vi "f1.vi"() -> ()   [LabVIEW 2020]
uses:
  <vilib>/MakerHub/LINX/Public/Peripherals/Analog/Analog Read 1 Chan.vi
  <vilib>/MakerHub/LINX/Public/Peripherals/Digital/Digital Write 1 Chan.vi
  <vilib>/MakerHub/LINX/Public/Peripherals/Analog/Analog Read N Chans.vi
  <vilib>/MakerHub/LINX/Public/Peripherals/Digital/Digital Write N Chans.vi
  <vilib>/MakerHub/LINX/Private/Local IO/LinxAnalogRead.vi
  <vilib>/MakerHub/LINX/Public/Utilities/Check Channel.vi
  <vilib>/MakerHub/LINX/Private/Local IO/LinxDigitalWrite.vi
  <vilib>/MakerHub/LINX/Public/Utilities/Open Serial.vi
  <vilib>/MakerHub/LINX/Private/Utilties/Generate Error.vi
  <vilib>/MakerHub/LINX/LMH-LINX.lvlib
panel:
  out "Voltage":dbl
  in  "stop":bool
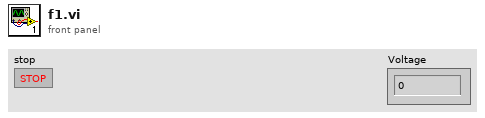
[diagram p1: front panel]
types:
  T1 = typedef "LMH-LINX.lvlib/LINX Ref.ctl" = cluster{"IO":T2, "Interface":T3, "LINX Device Config":T4}
  T2 = typedef "LMH-LINX.lvlib/Platform.ctl" = enum16{"Remote", "Local"}
  T3 = typedef "LMH-LINX.lvlib/Interface.ctl" = enum16{"Serial", "TCP"}
  T4 = typedef "LMH-LINX.lvlib/Device.lvlib/LINX Device Config.ctl" = cluster{"Interface":T3, "COM Port":refnum<visa-resource-name>, "TCP Configuration":T5, "Device Family":u8, "Device ID":u8, "Device Name":string, "TCP Ref":refnum<k5>, "Channels":T6}
  T5 = typedef "LMH-LINX.lvlib/Device.lvlib/TCP Config.ctl" = cluster{"IP Address":string, "Port":u16}
  T6 = typedef "LMH-LINX.lvlib/Channels.ctl" = cluster{"DI":u8[], "DO":u8[], "AI":u8[], "AO":u8[], "PWM":u8[], "QE":u8[], "UART":u8[], "I2C 2":u8[], "SPI":u8[], "CAN":u8[], "Servo":u8[], "AI Ref (V)":dbl, "AI Resolution (Bits)":u8, "AO Ref (V)":dbl, "AO Resolution (Bits)":u8}
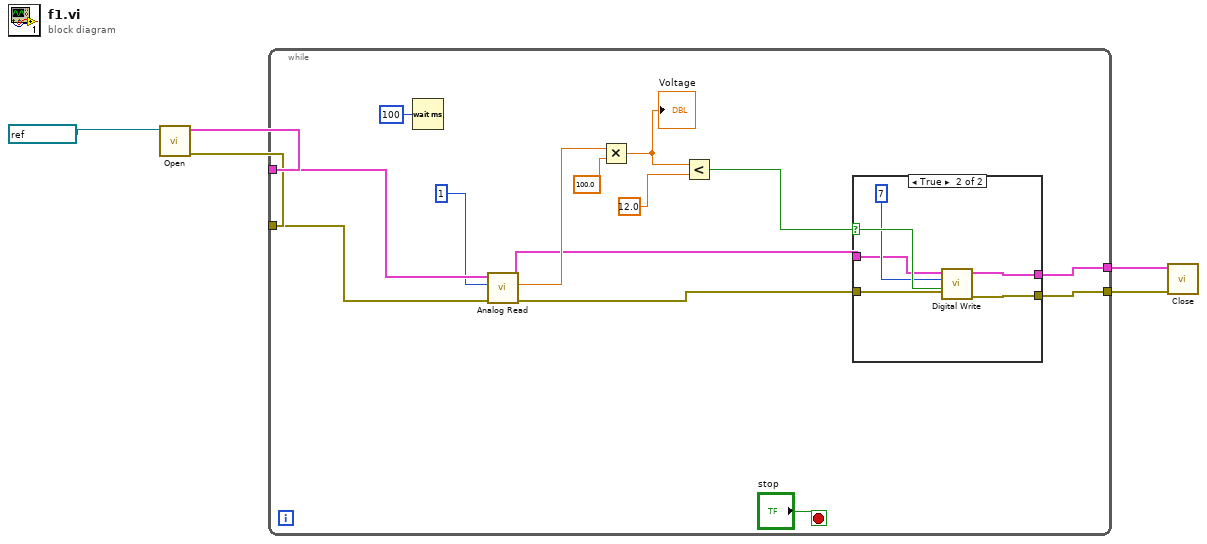
[diagram p0: block diagram]
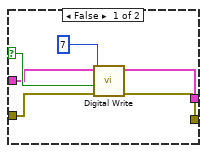
[diagram p2: hidden frame]
diagram:
  n1 = call-poly <vilib>:"Open.vi"("Serial Port"=refnum<visa-resource-name> "COM13") -> ("Error Out"=w4:errorcluster, "LINX Resource"=w5:T1)  [unwired: 8 in, 1 out]
  n2 = while {
    tunnel: w5 -> [w19]
    tunnel: w4 -> [w18]
    tunnel: [w11] -> w2
    tunnel: [w10] -> w1
    stop <- "stop" stop-if-true
    n3 = Wait (ms)(milliseconds to wait=u32 100) -> ()  [unwired: 1 out]
    n4 = call-poly <vilib>:"Analog Read.vi"("Error In"=w18, "Analog Channel"=u8 1, "LINX Resource"=w19) -> ("Error Out"=w9:errorcluster, "Voltage"=w13:dbl, "LINX Resource"=w12:T1)  [unwired: 5 in, 1 out]
    n5 = Multiply(x=w13, y=100.0) -> (x*y=w8:dbl)
    "Voltage" <- w8
    n6 = Less?(x=w8, y=12.0) -> (x < y?=w6:bool)
    n7 = case shown="True" w6 {
      selector: w6 -> [w23 w29]
      tunnel: [w25 w31] -> w10
      tunnel: [w24 w30] -> w11
      tunnel: w12 -> [w21 w27]
      tunnel: w9 -> [w20 w26]
      frame False {
        n8 = call-poly <vilib>:"Digital Write.vi"("Error In"=w20, "Output Value"=w23, "DO Channel"=u8 7, "LINX Resource"=w21) -> ("Error Out"=w24:errorcluster, "LINX Resource"=w25:T1)  [unwired: 6 in]
      }
      frame True {
        n9 = call-poly <vilib>:"Digital Write.vi"("Error In"=w26, "Output Value"=w29, "DO Channel"=u8 7, "LINX Resource"=w27) -> ("Error Out"=w30:errorcluster, "LINX Resource"=w31:T1)  [unwired: 6 in]
      }
    }
  }
  n10 = call <vilib>:"Close.vi"("Error In"=w2, "LINX Resource"=w1) -> ()  [unwired: 9 in, 1 out]
